vi "Shooter Teleop.vi"(11 "POVs":i16[](array[numeric])) -> ()   [LabVIEW 2020]
uses:
  Shooter/Sub-VI/Shooting Mode.ctl
  <vilib>/Rock Robotics/Network Tables/NT Read Number.vi
  <vilib>/Rock Robotics/Network Tables/NT Write Number.vi
  <vilib>/Rock Robotics/Network Tables/NT Write Boolean.vi
panel:
  out "Distance":dbl
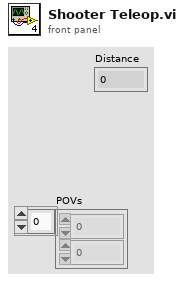
[diagram p1: front panel]
types:
  T1 = typedef "Shooting Mode.ctl" = enum16{"low", "high"}
  T2 = cluster{"Limelight Distance Constants":cluster{"angle of limelight":dbl, "height of top hub - height of limelight":dbl, "offset between true distance and distance from bumper to hub":dbl}, "Preset Ranges":cluster{"angle of limelight":dbl, "height of top hub - height of limelight":dbl}[], "Shooter Table":dbl[][]}
  T3 = cluster{"angle of limelight":dbl, "height of top hub - height of limelight":dbl, "offset between true distance and distance from bumper to hub":dbl}
  T4 = cluster{"low flywheel":dbl, "high flywheel":dbl, "hood":dbl}
  T5 = cluster{"hood":dbl, "Numeric":dbl, "top flywheel":dbl}
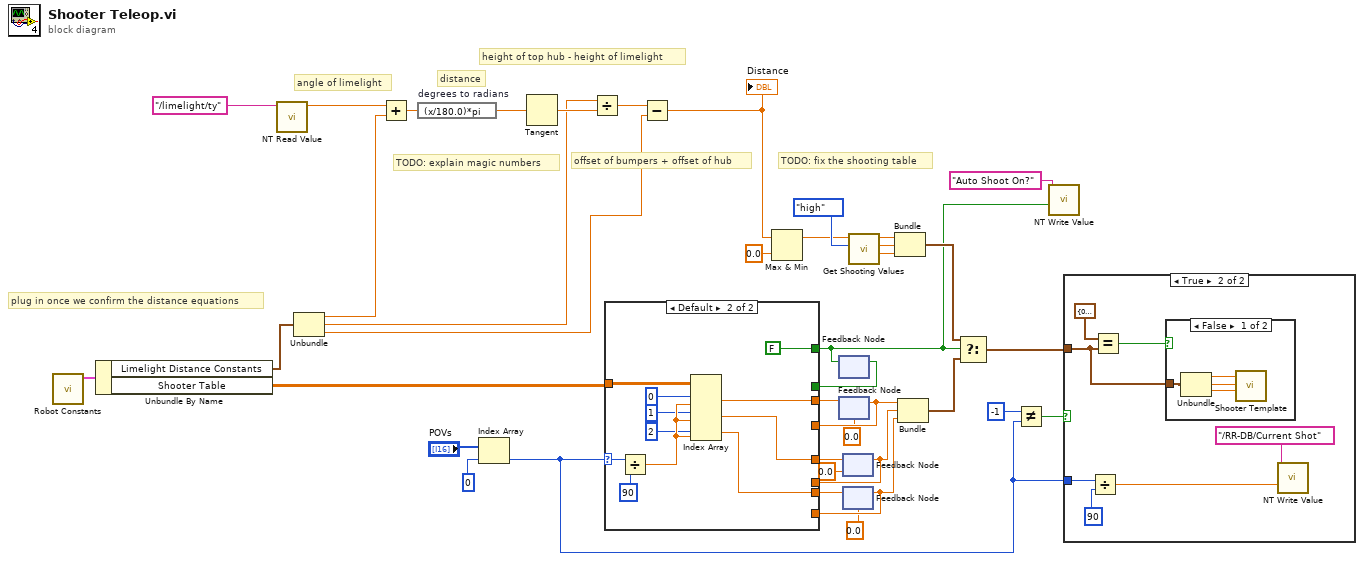
[diagram p0: block diagram]
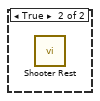
[diagram p3: hidden frame]
diagram:
  # "plug in once we confirm the distance equations"
  # "TODO: fix the shooting table"
  # "offset of bumpers + offset of hub"
  # "height of top hub - height of limelight"
  # "angle of limelight"
  # "TODO: explain magic numbers"
  # "distance"
  n1 = call "Robot Constants.vi"() -> ("Robot Data"=w11:T2)  [unwired: 11 in]
  n2 = Unbundle By Name(w11) -> ("Limelight Distance Constants"=w10:T3, "Shooter Table"=w9:dbl[][])
  n3 = call-poly <vilib>:"NT Read Value.vi"("Name"="/limelight/ty") -> ("Numeric"=w38:dbl)  [unwired: 9 in, 1 out]
  n4 = Unbundle(w10) -> ("angle of limelight"=w6:dbl, "height of top hub - height of limelight"=w5:dbl, "offset between true distance and distance from bumper to hub"=w4:dbl)
  n5 = Add(x=w38, y=w6) -> (x+y=w36:dbl)
  n6 = expression code="(x/180.0)*pi" "degrees to radians"(w36) -> (w35:dbl)
  n7 = Index Array(array="POVs", index=0) -> (element=w8:i16)
  n8 = Tangent(1:w35) -> (0:w37:dbl)
  n9 = Divide(x=w5, y=w37) -> (x/y=w34:dbl)
  n10 = Subtract(x=w34, y=w4) -> (x-y=w12:dbl)
  "Distance" <- w12
  n11 = Max & Min(x=w12, y=0.0) -> (max(x,y)=w24:dbl)  [unwired: 1 out]
  n12 = feedback #1() -> (w28:bool)  [unwired: 1 in]
  n13 = feedback #2(0.0) -> (w27:dbl)
  n14 = feedback #3(0.0) -> (w26:dbl)
  n15 = feedback #4(0.0) -> (w25:dbl)
  n16 = case shown="Default" w8 {
    selector: w8 -> [_ w48]
    tunnel: [w43 w52] -> w30
    tunnel: [w42 w51] -> w16
    tunnel: [w41 w50] -> w29
    tunnel: [w40 FALSE] -> w13
    tunnel: w27 -> [w43 _]
    tunnel: w26 -> [w42 _]
    tunnel: w25 -> [w41 _]
    tunnel: w28 -> [w40 _]
    tunnel: w9 -> [_ w53]
    frame -1 {
    }
    frame Default {
      n17 = Divide(x=w48, y=90) -> (x/y=w47:dbl)
      n18 = Index Array(array=w53, index (row) #1=0 ("disabled index (row)"), index (col) #1=w47, index (row) #2=1 ("disabled index (row)"), index (col) #2=w47, index (row) #3=2 ("disabled index (row)"), index (col) #3=w47) -> (element #1=w52:dbl, element #2=w51:dbl, element #3=w50:dbl)
    }
  }
  n19 = feedback-in #1(w13) -> ()
  n20 = feedback-in #2(w30) -> ()
  n21 = feedback-in #3(w16) -> ()
  n22 = feedback-in #4(w29) -> ()
  n23 = call "Get Shooting Values.vi"("Shooting Mode"=Shooting_Mode."high", "distance"=w24) -> ("hood"=w21:dbl, "high flywheel"=w22:dbl, "low flywheel"=w23:dbl)  [unwired: 7 in]
  n24 = Bundle("low flywheel"=w23, "high flywheel"=w22, "hood"=w21) -> (w20:T4)  [unwired: 1 in]
  n25 = Bundle(w27, w26, w25) -> (w7:cluster{dbl, dbl, dbl})  [unwired: 1 in]
  n26 = Select(t=w20, s=w13, f=w7) -> (s? t:f=w19:T4)
  n27 = Not Equal?(x=i16 -1, y=w8) -> (x != y?=w14:bool)
  n28 = call-poly <vilib>:"NT Write Value.vi"("Boolean"=w13, "Name"="Auto Shoot On?") -> ()  [unwired: 9 in, 1 out]
  n29 = case shown="True" w14 {
    tunnel: w19 -> [_ w61]
    tunnel: w8 -> [_ w57]
    frame False {
    }
    frame True {
      n30 = Divide(x=w57, y=90) -> (x/y=w55:dbl)
      n31 = Equal?(x=T5 {"hood"=0.0, "Numeric"=0.0, "top flywheel"=0.0}, y=w61) -> (x = y?=w59:bool)
      n32 = case shown="False" w59 {
        tunnel: w61 -> [w65 _]
        frame False {
          n33 = Unbundle(w65) -> ("low flywheel"=w64:dbl, "high flywheel"=w63:dbl, "hood"=w62:dbl)
          n34 = call "Shooter Template.vi"("top flywheel (vol)"=w62, "flywheel (vol)"=w63, "hood (pos)"=w64) -> ()  [unwired: 8 in, 1 out]
        }
        frame True {
          n35 = call "Shooter Rest.vi"() -> ()  [unwired: 11 in, 1 out]
        }
      }
      n36 = call-poly <vilib>:"NT Write Value.vi"("Numeric"=w55, "Name"="/RR-DB/Current Shot") -> ()  [unwired: 9 in, 1 out]
    }
  }
